vi "ATDome_logEvent_shutterInPosition.vi"(8 "error in (no error)":errorcluster, 11 "logevent_shutterInPosition_Ctl":T1) -> (0 "error out":errorcluster, 2 "function return":i32, 3 "logevent_shutterInPosition_Ctl out":T1)   [LabVIEW 2016, in "SALLV_ATDome.lvlib"]
doc: "int ATDome_shm_logEvent_shutterInPositionLV(ATDome_logevent_shutterInPositionLV *logevent_shutterInPosition_Ctl );"
uses:
  SALLV_ATDome.lvlib
  DataTypes/logevent_shutterInPosition.ctl
  SALLV_ATDome.so
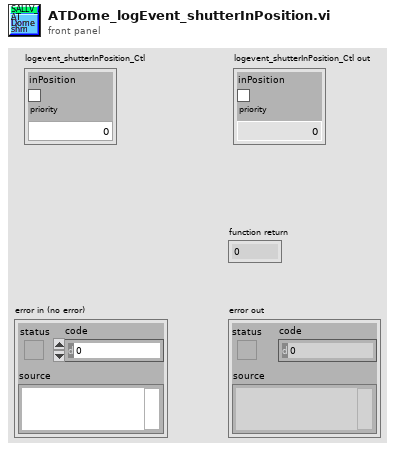
[diagram p1: front panel]
types:
  T1 = typedef "SALLV_ATDome.lvlib/logevent_shutterInPosition.ctl" = cluster{"inPosition":bool, "priority":i32}
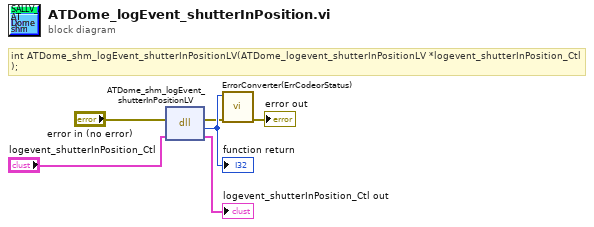
[diagram p0: block diagram]
diagram:
  # "int ATDome_shm_logEvent_shutterInPositionLV(ATDome_logevent_shutterInPositionLV *logevent_shutterInPosition_Ctl );"
  n1 = dll-call lib="home/andres/Desktop/SAL_ATDome/SALLV_ATDome.*" fn="ATDome_shm_logEvent_shutterInPositionLV"(error in="error in (no error)", "logevent_shutterInPosition_Ctl"="logevent_shutterInPosition_Ctl") -> (error out=w2:errorcluster, w6:i32, "logevent_shutterInPosition_Ctl"=→"logevent_shutterInPosition_Ctl out":T1)  [unwired: 2 in, 1 out]
  "function return" <- w6
  n2 = call "ErrorConverter(ErrCodeorStatus).vi"("error in (no error)"=w2, "error code"=w6) -> ("error out"=→"error out":errorcluster)  [unwired: 9 in]
